vi "KE622x -- Set Current Range.vi"(0 "Resource In":refnum<visa-resource-name>, 1 "Check For SCPI Errors? (T)":bool=TRUE, 7 "Current Range":T1, 11 "error in (no error)":errorcluster) -> (4 "Resource Out (dupl)":refnum<visa-resource-name>, 15 "error out":errorcluster)   [LabVIEW 2013, in "Keithly user program.lvlib"]
doc: "Allows the user to either auto-select the current range based on the current level, or manually specify a range."
uses:
  Keithly user program.lvlib
  Typedefs/KE622x -- Current Range.ctl
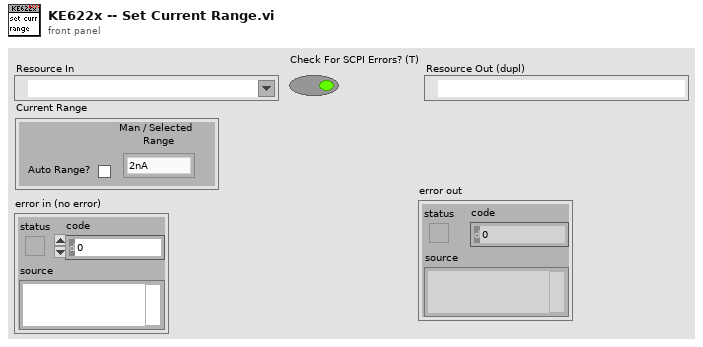
[diagram p1: front panel]
types:
  T1 = typedef "Keithly user program.lvlib/KE622x -- Current Range.ctl" = cluster{"Auto Range?":bool, "Man / Selected\n        Range":enum16{"2nA", "20nA", "200nA", "2uA", "20uA", "200uA", "2mA", "20mA", "100mA"}}
  T2 = enum16{"2nA", "20nA", "200nA", "2uA", "20uA", "200uA", "2mA", "20mA", "100mA"}
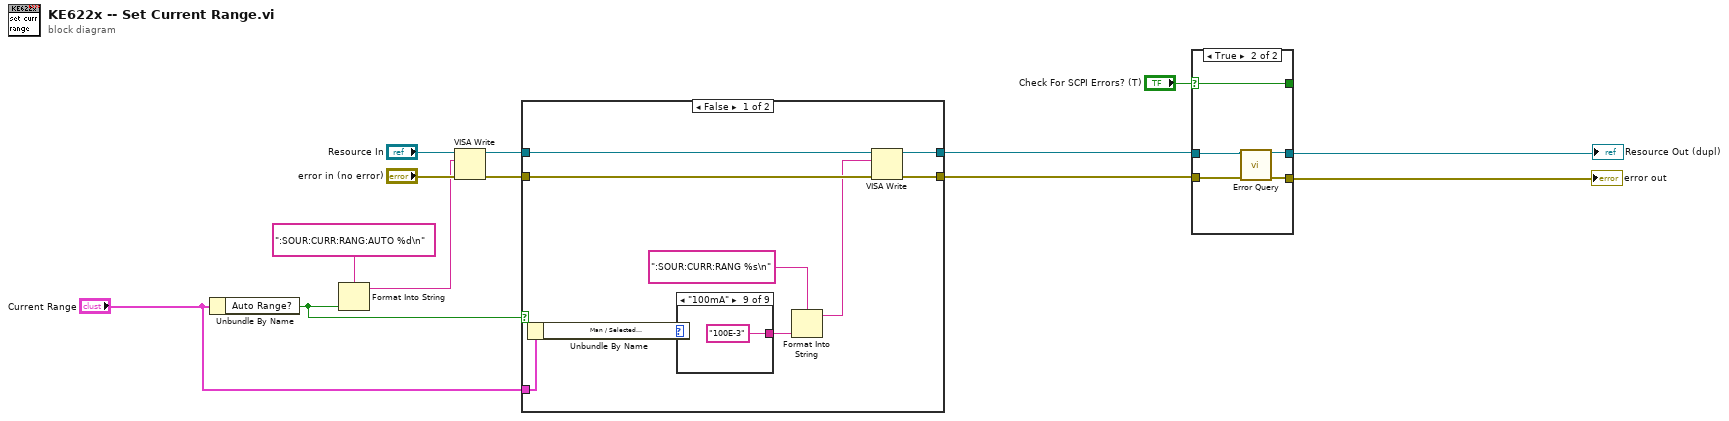
[diagram p0: block diagram]
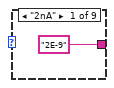
[diagram p2: hidden frame]
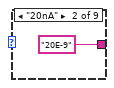
[diagram p3: hidden frame]
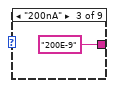
[diagram p4: hidden frame]
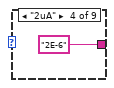
[diagram p5: hidden frame]
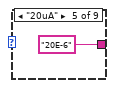
[diagram p6: hidden frame]
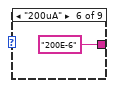
[diagram p7: hidden frame]
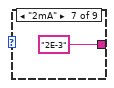
[diagram p8: hidden frame]
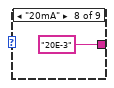
[diagram p9: hidden frame]
diagram:
  n1 = Unbundle By Name("Current Range") -> ("Auto Range?"=w6:bool)
  n2 = Format Into String(format string=":SOUR:CURR:RANG:AUTO %d\n", w6) -> (resulting string=w9:string)  [unwired: 2 in, 1 out]
  n3 = VISA Write(VISA resource name="Resource In", write buffer=w9, error in (no error)="error in (no error)") -> (VISA resource name out=w8:refnum<visa-resource-name>, error out=w7:errorcluster)  [unwired: 1 out]
  n4 = case shown="False" w6 {
    tunnel: w8 -> [w22 w33]
    tunnel: w7 -> [w21 w32]
    tunnel: "Current Range" -> [w14 _]
    tunnel: [w16 w32] -> w4
    tunnel: [w15 w33] -> w5
    frame False {
      n5 = Unbundle By Name(w14) -> ("Man / Selected\n        Range"=w20:T2)
      n6 = case shown="\"100mA\"" w20 {
        tunnel: ["2E-9" "20E-9" "200E-9" "2E-6" "20E-6" "200E-6" "2E-3" "20E-3" "100E-3"] -> w18
        frame "2nA" {
        }
        frame "20nA" {
        }
        frame "200nA" {
        }
        frame "2uA" {
        }
        frame "20uA" {
        }
        frame "200uA" {
        }
        frame "2mA" {
        }
        frame "20mA" {
        }
        frame "100mA" {
        }
      }
      n7 = Format Into String(format string=":SOUR:CURR:RANG %s\n", w18) -> (resulting string=w17:string)  [unwired: 2 in, 1 out]
      n8 = VISA Write(VISA resource name=w22, write buffer=w17, error in (no error)=w21) -> (VISA resource name out=w15:refnum<visa-resource-name>, error out=w16:errorcluster)  [unwired: 1 out]
    }
    frame True {
    }
  }
  n9 = case shown="True" "Check For SCPI Errors? (T)" {
    selector: "Check For SCPI Errors? (T)" -> [w34 w41]
    tunnel: w5 -> [w36 w40]
    tunnel: w4 -> [w35 w39]
    tunnel: [w35 w37] -> w2
    tunnel: [w36 w38] -> w3
    tunnel: [w34 w41] -> _
    frame False {
    }
    frame True {
      n10 = call "Error Query.vi"("VISA Resource In"=w40, "error in (no error)"=w39) -> ("VISA Resource Out (dupl)"=w38:refnum<visa-resource-name>, "error out"=w37:errorcluster)  [unwired: 10 in, 2 out]
    }
  }
  "Resource Out (dupl)" <- w3
  "error out" <- w2
